vi "GH-311.vi"(8 "Error In":errorcluster, 10 "SIG Pin (DIO)":u8, 11 "LINX Resource":T1) -> (0 "Error Out":errorcluster, 1 "Inches":dbl, 2 "Centimeters":dbl, 3 "LINX Resource":T1)   [LabVIEW 2011, in "LMH-LINX.lvlib" / "Ultrasonic.lvlib"]
doc: "Read distance using the GH-311 ultrasonic distance sensor."
uses:
  Ultrasonic.lvlib
  Private/Type Defs/LINX Ref.ctl
  Private/Type Defs/Platform.ctl
  Private/Type Defs/Interface.ctl
  Private/Device/Type Defs/LINX Device Config.ctl
  Private/Device/Type Defs/TCP Config.ctl
  Private/Device/Type Defs/Channels.ctl
  LMH-LINX.lvlib
  Private/Device/Device.lvlib
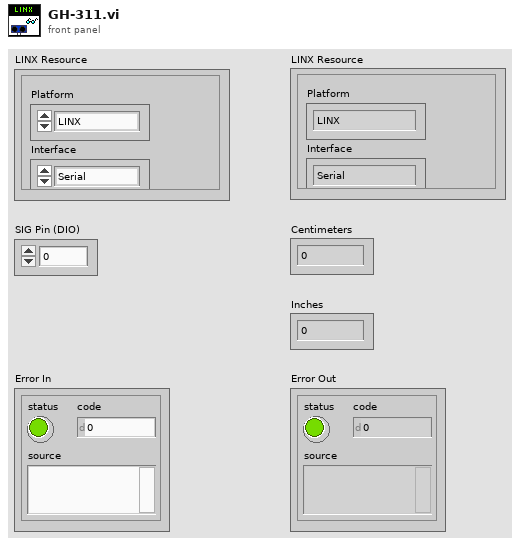
[diagram p1: front panel]
types:
  T1 = typedef "LMH-LINX.lvlib/LINX Ref.ctl" = cluster{"Platform":T2, "Interface":T3, "LINX Device Config":T4}
  T2 = typedef "LMH-LINX.lvlib/Platform.ctl" = enum16{"LINX", "myRIO"}
  T3 = typedef "LMH-LINX.lvlib/Interface.ctl" = enum16{"Serial", "TCP"}
  T4 = typedef "LMH-LINX.lvlib/Device.lvlib/LINX Device Config.ctl" = cluster{"Interface":T3, "COM Port":refnum<visa-resource-name>, "TCP Configuration":T5, "Device Family":u8, "Device ID":u8, "Device Name":string, "TCP Ref":refnum<k5>, "Channels":T6}
  T5 = typedef "LMH-LINX.lvlib/Device.lvlib/TCP Config.ctl" = cluster{"IP Address":string, "Port":u16}
  T6 = typedef "LMH-LINX.lvlib/Channels.ctl" = cluster{"DI":u8[], "DO":u8[], "AI":u8[], "AO":u8[], "PWM":u8[], "QE":u8[], "UART":u8[], "I2C 2":u8[], "SPI":u8[], "CAN":u8[], "Servo":u8[], "AI Ref (V)":dbl, "AO Ref (V)":dbl, "AO Resolution (Bits)":u8}
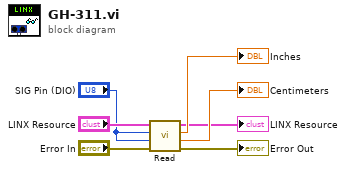
[diagram p0: block diagram]
diagram:
  n1 = call "Read.vi"("Error In"="Error In", "DO Channel"="SIG Pin (DIO)", "DI Channel"="SIG Pin (DIO)", "LINX Resource"="LINX Resource") -> ("Error Out"=→"Error Out":errorcluster, "Centimeters"=→"Centimeters":dbl, "Inches"=→"Inches":dbl, "LINX Resource"=→"LINX Resource":T1)  [unwired: 4 in]
